vi "Init Message Queue.vi"(8 "error in (no error)":errorcluster) -> (0 "error out":errorcluster, 3 "Queue out":refnum<queue>)   [LabVIEW 2020, in "Debugger.lvclass"]
uses:
  Debugger.lvclass
  Debugger.lvclass/Debugger.ctl
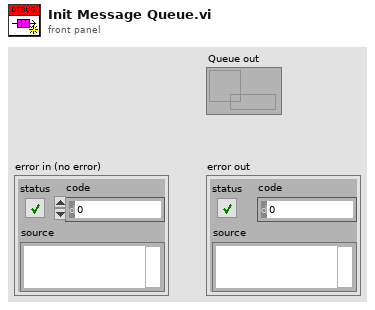
[diagram p1: front panel]
types:
  T1 = cluster{"Message":string, "Message Data":variant}
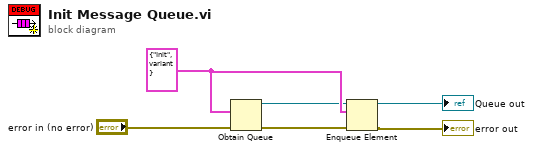
[diagram p0: block diagram]
diagram:
  w2 = T1 {"Message"="Init", "Message Data"=variant} ("Message Cluster")
  n1 = Obtain Queue(element data type=w2, error in (no error)="error in (no error)") -> (queue out=w1:refnum<queue>, error out=w6:errorcluster)  [unwired: 3 in, 1 out]
  n2 = Enqueue Element(queue=w1, element=w2, error in (no error)=w6) -> (queue out=→"Queue out":refnum<queue>, error out=→"error out":errorcluster)  [unwired: 1 in, 1 out]
